vi "Timed Read from Hardware.vi"(8 "error in":errorcluster, 10 "Values in":dbl[](array[numeric]), 11 "Execution Unit in":refnum<class "Execution Unit.lvclass">) -> (0 "error out":errorcluster, 2 "Values out":dbl[](array[numeric]), 3 "Execution Unit out":refnum<class "Execution Unit.lvclass">)   [LabVIEW 2024, in "AIM ARINC 429 Engine.lvlib" / "Custom Device.lvlib"]
uses:
  Custom Device.lvlib
  Interfaces/Execution Unit/Execution Unit.lvclass
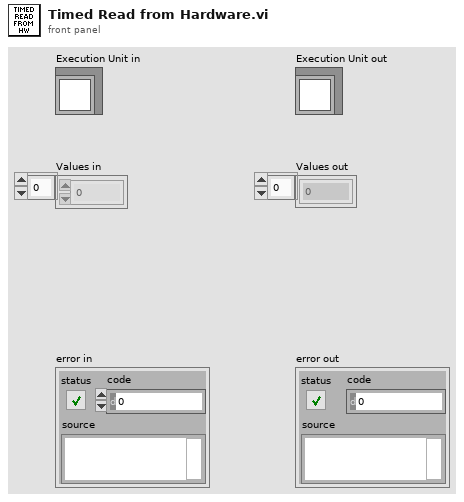
[diagram p1: front panel]
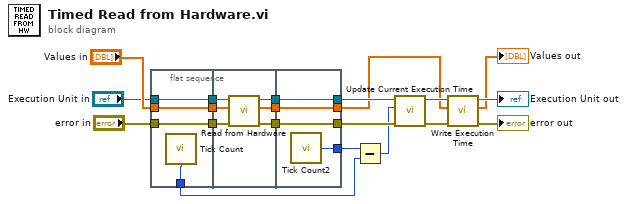
[diagram p0: block diagram]
diagram:
  n1 = flat-sequence {
    tunnel: "Values in" -> [w22]
    tunnel: "error in" -> [w23]
    tunnel: "Execution Unit in" -> [w24]
    tunnel: [w24] -> w20
    tunnel: [w23] -> w19
    tunnel: [w22] -> w18
    tunnel: [w21] -> w14
    tunnel: w20 -> [w28]
    tunnel: w19 -> [w27]
    tunnel: w18 -> [w26]
    tunnel: [w30] -> w17
    tunnel: [w29] -> w16
    tunnel: [w25] -> w15
    tunnel: [w32] -> w1
    tunnel: [w33] -> w5
    tunnel: [w34] -> w6
    tunnel: w17 -> [w34]
    tunnel: w16 -> [w33]
    tunnel: w15 -> [w32]
    tunnel: [w31] -> w13
    frame #0 {
      n2 = call "Tick Count"() -> ("Tick Count(uSec)"=w21:u32)
    }
    frame #1 {
      n3 = call-dynamic "Read from Hardware.vi"("error in (no error)"=w27, "Values in"=w26, "Execution Unit in"=w28) -> ("error out"=w30:errorcluster, "Values out"=w25:dbl[], "Execution Unit out"=w29:refnum<class "Execution Unit.lvclass">)  [unwired: 6 in]
    }
    frame #2 {
      n4 = call "Tick Count2"() -> ("Tick Count(uSec)"=w31:u32)
    }
  }
  n5 = Subtract(x=w13, y=w14) -> (x-y=w4:u32)
  n6 = call-dynamic "Update Current Execution Time.vi"("error in (no error)"=w6, "Current Execution Time (us)"=w4, "Execution Unit in"=w5) -> ("error out"=w3:errorcluster, "Execution Unit out"=w2:refnum<class "Execution Unit.lvclass">)  [unwired: 7 in]
  n7 = call-dynamic "Write Execution Time.vi"("error in (no error)"=w3, "Values in"=w1, "Execution Unit in"=w2) -> ("error out"=→"error out":errorcluster, "Values out"=→"Values out":dbl[], "Execution Unit out"=→"Execution Unit out":refnum<class "Execution Unit.lvclass">)  [unwired: 6 in]
